vi "Save Array to file and-or select new target file.vi"(9 "Choose New \nSave Target":bool, 10 "Save Results":bool, 11 "Values to Save":string[](array[string])) -> (3 "selected path":path)   [LabVIEW 2016]
uses:
  <vilib>/Utility/file.llb/Write Delimited Spreadsheet (string).vi
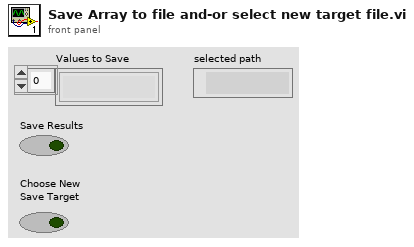
[diagram p1: front panel]
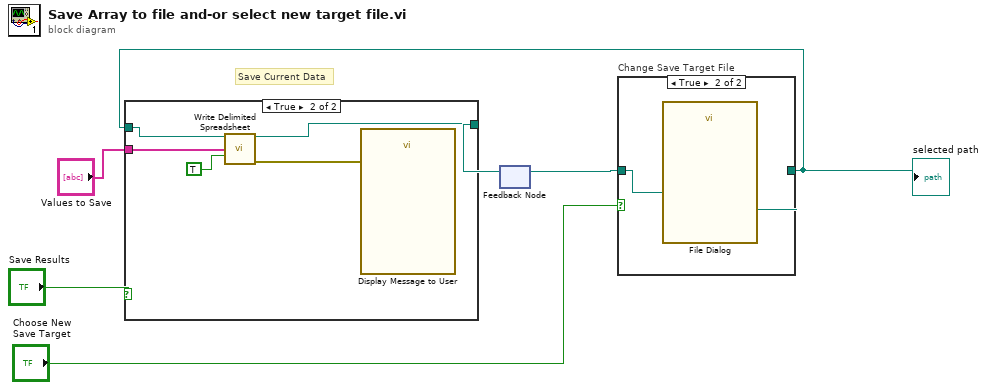
[diagram p0: block diagram]
diagram:
  # "Save Current Data"
  n1 = feedback #1() -> (w4:path)  [unwired: 1 in]
  n2 = case "Change Save Target File" shown="True" "Choose New \nSave Target" {
    tunnel: w4 -> [w7 w9]
    tunnel: [w7 w8] -> w5
    frame False {
    }
    frame True {
      n3 = call "File Dialog"("start path"=w9) -> ("selected path"=w8:path)  [unwired: 11 in, 3 out]
    }
  }
  "selected path" <- w5
  n4 = case shown="True" "Save Results" {
    tunnel: "Values to Save" -> [_ w15]
    tunnel: [w10 w12] -> w3
    tunnel: w5 -> [w10 w11]
    frame False {
    }
    frame True {
      n5 = call-poly <vilib>:"Write Delimited Spreadsheet.vi"("file path (dialog if empty)"=w11, "1D data"=w15, "append to file? (new file:F)"=TRUE ("append to file? (F)")) -> ("new file path (Not A Path if cancelled)"=w12:path, "error out"=w13:errorcluster)  [unwired: 11 in]
      n6 = call "Display Message to User"("error in (no error)"=w13) -> ()  [unwired: 9 in, 2 out]
    }
  }
  n7 = feedback-in #1(w3) -> ()
